vi "Write Iterations.vi"(10 "Iterations":u32, 11 "For Loop Dialog in":refnum<class "For Loop Dialog.lvclass">) -> (3 "For Loop Dialog out":refnum<class "For Loop Dialog.lvclass">)   [LabVIEW 2017, in "For Loop Dialog.lvclass"]
uses:
  <vilib>/gpm_packages/@cs/Test-executive-builder/Source/Test Executive Builder Dialogs/For Loop Dialog/For Loop Dialog.lvclass
  <vilib>/gpm_packages/@cs/Test-executive-builder/Source/Test Executive Builder Dialogs/For Loop Dialog/For Loop Dialog.lvclass/For Loop Dialog.ctl
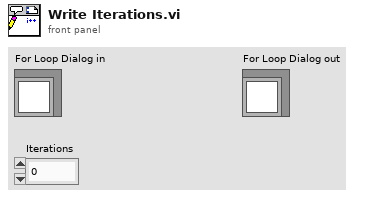
[diagram p1: front panel]
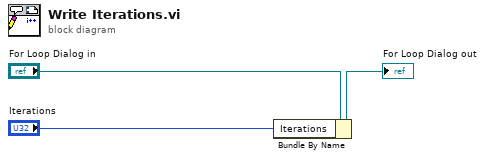
[diagram p0: block diagram]
diagram:
  n1 = Bundle By Name(cluster="For Loop Dialog in", "Iterations"="Iterations") -> (→"For Loop Dialog out":refnum<class "For Loop Dialog.lvclass">)
